vi "Behavior.vi"() -> ()   [LabVIEW 2014]
doc: "Use this template to measure or generate signals using the DAQ Assistant Express VI and NI-DAQmx. Double click the DAQ Assistant Express VI to launch a configuration wizard which steps you through configuring a measurement or generation.\n\nNote: You must have an NI-DAQmx compatible device installed to use this Express VI. Refer to the DAQ Quick Start Guide for NI-DAQ 7.0 for a list of compatible devices."
uses:
  <vilib>/userdefined/High Color/IMAQdx.ctl
  QuadraturePositionDecoder/QuadraturePositionDecoder.lvclass
  Imaging/Imaging.lvclass
  Photodiode/Photodiode.lvclass
panel:
  in  "Analog Signals":bool=TRUE
  in  "Ball Motion":bool=TRUE
  in  "Video":bool=TRUE
  in  "Base path":path
  out "Waveform Chart":dynamicdata(graph)
  in  "Remote":bool
  out "Scanning":bool
  out "Recording":bool
  out "File":path
  in  "Rec":bool
  out "File Path":path
  in  "Save Analog Signals":bool=TRUE
  out "Ball Position":u32
  in  "Compression":string(combo)="None"
  in  "Save Ball Motion":bool=TRUE
  in  "Save Video":bool=TRUE
  in  "Gain":dbl(slide)=2.6607250597988097 min=1.0 max=3.9810717055349722 scale=0.0..4.0
  in  "Exposure":dbl(slide)=16602.0 caption="Exposure Time" min=0.0 max=50000.0 scale=16.6..50000.0 scale format="%#_2p"
  out "FPS":dbl format="%#.0f"
  in  "Fps":i32=20
  out "Video Frames":T1(plugin-control)
  out "Ball Speed":dbl(graph)
  out "Stopped":bool
  in  "Stop":bool
  # "TODO:\n1. Make EyeParams me properly set\n2. Synchronization"
  # "Hardware Used For Quadrature Decoding"
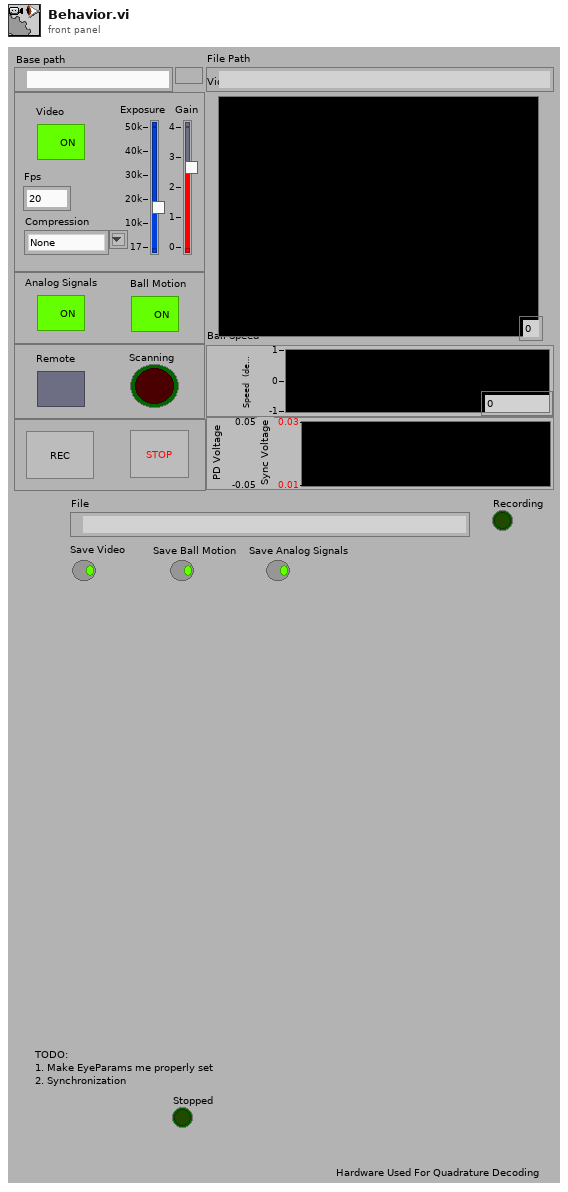
[diagram p1: front panel]
types:
  T1 = typedef "IMAQ Image.ctl" = refnum<image>
  T2 = typedef "IMAQdx.ctl" = refnum<k21>
  T3 = cluster{"VISA resource name":refnum<visa-resource-name>, "Counter":tag, "A Input Terminal":tag, "B Input Terminal":tag, "Z Index Terminal":tag, "Camera Name":T2, "Timestamp Counter":tag, "Timestamp Source":tag, "photodiode":tag, "scanimageframesync":tag, "Default Path":string}[]
  T4 = cluster{"VISA resource name":refnum<visa-resource-name>, "Counter":tag, "A Input Terminal":tag, "B Input Terminal":tag, "Z Index Terminal":tag, "Camera Name":T2, "Timestamp Counter":tag, "Timestamp Source":tag, "photodiode":tag, "scanimageframesync":tag, "Default Path":string}
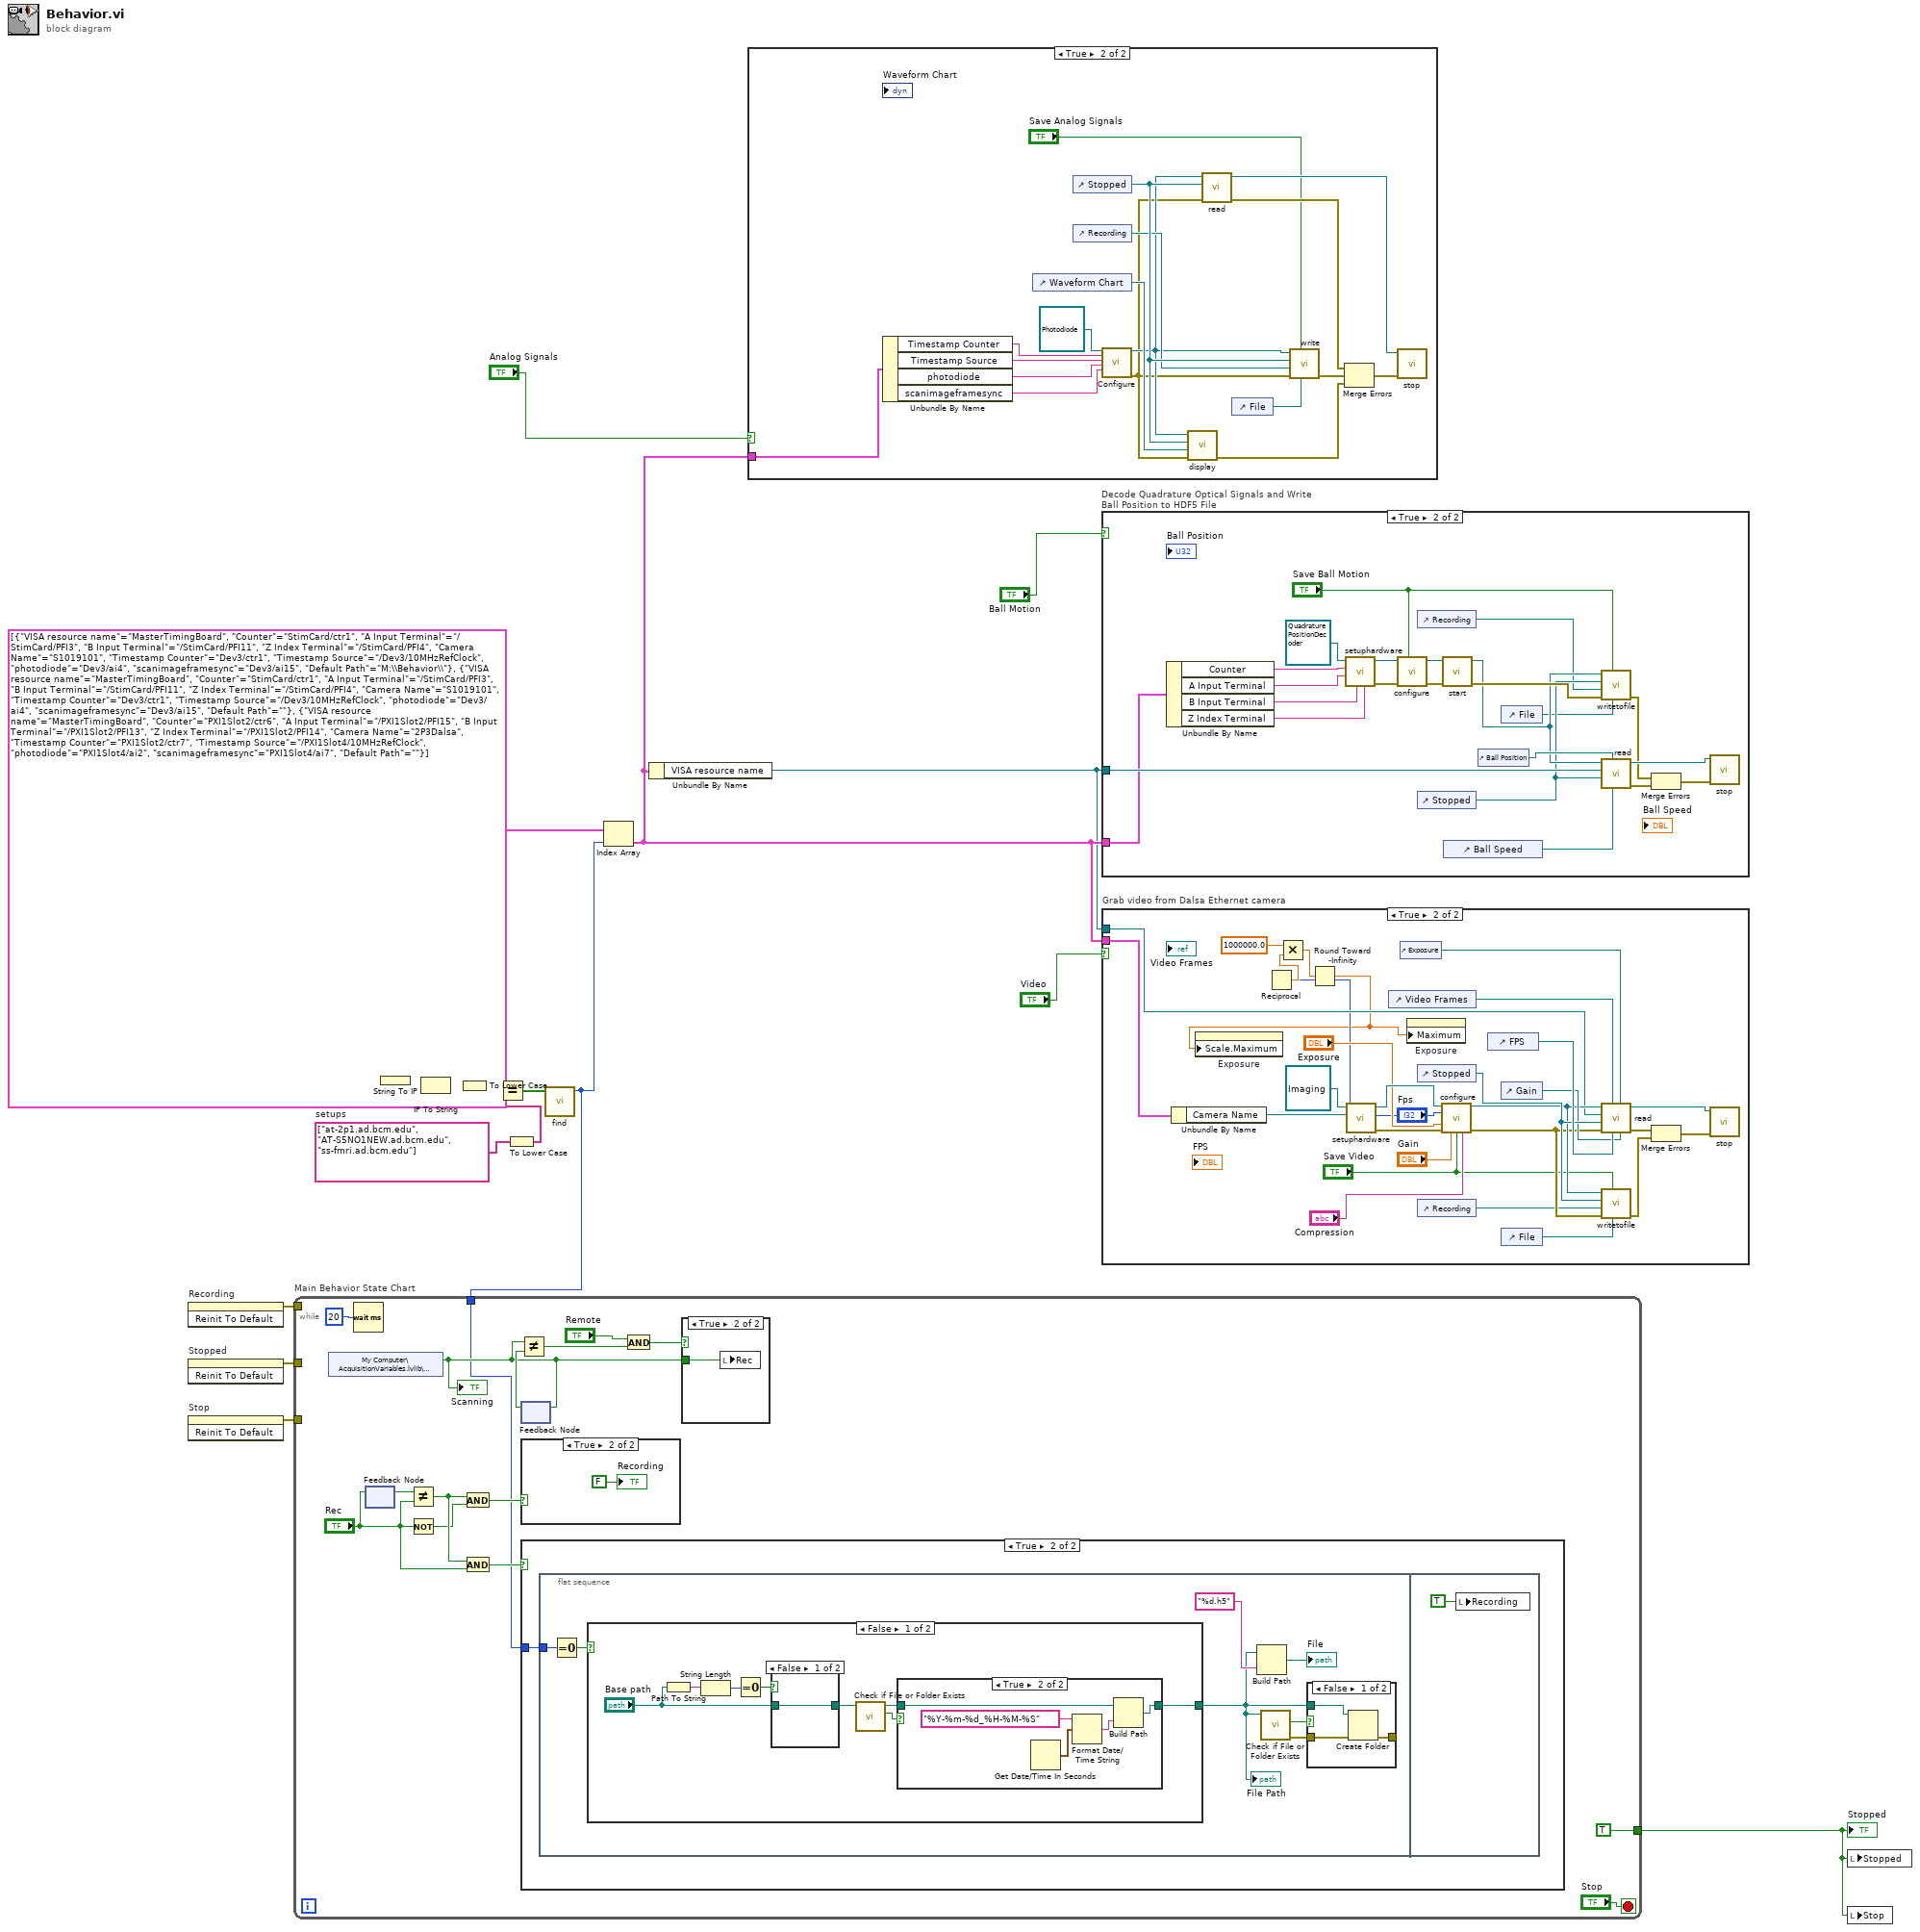
[diagram p0: block diagram]
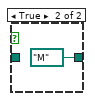
[diagram p8: hidden frame]
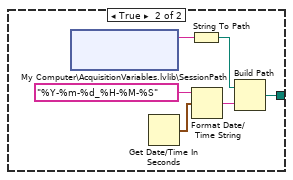
[diagram p10: hidden frame]
diagram:
  w3 = string[] ["at-2p1.ad.bcm.edu", "AT-S5NO1NEW.ad.bcm.edu", "ss-fmri.ad.bcm.edu"]  # setups
  n1 = invoke on="Recording" class="Bool (strict)" method="Reinit To Default"() -> (error out=w14:errorcluster)  [unwired: 3 in, 2 out]
  n2 = invoke on="Stopped" class="Bool (strict)" method="Reinit To Default"() -> (error out=w16:errorcluster)  [unwired: 3 in, 2 out]
  n3 = invoke on="Stop" class="Bool (strict)" method="Reinit To Default"() -> (error out=w17:errorcluster)  [unwired: 3 in, 2 out]
  n4 = String To IP() -> (0:w11:u32)  [unwired: 1 in]
  n5 = IP To String(2:w11) -> (0:w10:string)  [unwired: 1 in]
  n6 = To Lower Case(string=w10) -> (all lower case string=w9:string)
  n7 = To Lower Case(string=w3) -> (all lower case string=w2:string[])
  n8 = Equal?(x=w9, y=w2) -> (x = y?=w8:bool[])
  n9 = call "find.vi"("Array"=w8) -> ("Index"=w4:i32)  [unwired: 10 in]
  n10 = while "Main Behavior State Chart" {
    tunnel: [TRUE] -> w15
    tunnel: w17 -> [_]
    tunnel: w16 -> [_]
    tunnel: w14 -> [_]
    tunnel: w4 -> [w18]
    stop <- "Stop" stop-if-true
    n11 = shared-variable "My Computer\\AcquisitionVariables.lvlib\\AODScanning"() -> (w22:bool)  [unwired: 1 in, 1 out]
    "Scanning" <- w22
    n12 = Wait (ms)(milliseconds to wait=u32 20) -> ()  [unwired: 1 out]
    n13 = feedback-in #1("Rec") -> ()
    n14 = feedback #1() -> (w29:bool)  [unwired: 1 in]
    n15 = Not Equal?(x=w29, y="Rec") -> (x != y?=w27:bool)
    n16 = Not(x="Rec") -> (.not. x?=w26:bool)
    n17 = And(x=w27, y=w26) -> (x .and. y?=w24:bool)
    n18 = And(x=w27, y="Rec") -> (x .and. y?=w28:bool)
    n19 = feedback-in #2(w22) -> ()
    n20 = feedback #2() -> (w23:bool)  [unwired: 1 in]
    n21 = Not Equal?(x=w22, y=w23) -> (x != y?=w21:bool)
    n22 = case shown="True" w24 {
      frame False {
      }
      frame True {
        "Recording" <- FALSE
      }
    }
    n23 = case shown="True" w28 {
      tunnel: w18 -> [_ w35]
      frame False {
      }
      frame True {
        n24 = flat-sequence {
          tunnel: w35 -> [w38]
          frame #0 {
            n25 = Equal To 0?(x=w38) -> (x = 0?=w37:bool)
            n26 = case shown="False" w37 {
              tunnel: [w48 w60] -> w36
              frame False {
                n27 = Path To String(path="Base path") -> (string=w47:string)
                n28 = String Length(string=w47) -> (length=w46:i32)
                n29 = Equal To 0?(x=w46) -> (x = 0?=w45:bool)
                n30 = case shown="False" w45 {
                  tunnel: "Base path" -> [w51 _]
                  tunnel: [w51 path "M:/" ("Base path")] -> w43
                  frame False {
                  }
                  frame True {
                  }
                }
                n31 = call <vilib>:"Check if File or Folder Exists.vi"("path"=w43) -> ("file or folder exists?"=w49:bool, "dup path"=w50:path)  [unwired: 8 in, 1 out]
                n32 = case shown="True" w49 {
                  tunnel: w50 -> [w53 w56]
                  tunnel: [w53 w55] -> w48
                  frame False {
                  }
                  frame True {
                    n33 = Get Date/Time In Seconds() -> (seconds since 1Jan1904=w57:timestamp)
                    n34 = Format Date/Time String(time format string (%c)="%Y-%m-%d_%H-%M-%S", seconds (now)=w57) -> (date/time string=w58:string)  [unwired: 1 out]
                    n35 = Build Path(base path=w56, name or relative path=w58) -> (appended path=w55:path)
                  }
                }
              }
              frame True {
                n36 = shared-variable "My Computer\\AcquisitionVariables.lvlib\\SessionPath"() -> (w64:string)  [unwired: 2 in, 3 out]
                n37 = Get Date/Time In Seconds() -> (seconds since 1Jan1904=w63:timestamp)
                n38 = String To Path(string=w64) -> (path=w61:path)
                n39 = Format Date/Time String(time format string (%c)="%Y-%m-%d_%H-%M-%S", seconds (now)=w63) -> (date/time string=w62:string)  [unwired: 1 out]
                n40 = Build Path(base path=w61, name or relative path=w62) -> (appended path=w60:path)
              }
            }
            "File Path" <- w36
            n41 = Build Path(base path=w36, name or relative path="%d.h5" ("string")) -> (appended path=→"File":path)
            n42 = call <vilib>:"Check if File or Folder Exists.vi"("path"=w36) -> ("error out"=w40:errorcluster, "file or folder exists?"=w39:bool)  [unwired: 8 in, 1 out]
            n43 = case shown="False" w39 {
              tunnel: w36 -> [w67 _]
              tunnel: w40 -> [w66 w68]
              tunnel: [w65 w68] -> _
              frame False {
                n44 = Create Folder(path (use dialog)=w67, error in=w66) -> (error out=w65:errorcluster)  [unwired: 1 in, 2 out]
              }
              frame True {
              }
            }
          }
          frame #1 {
            n45 = local write "Recording"(TRUE) -> ()
          }
        }
      }
    }
    n46 = And(x="Remote", y=w21) -> (x .and. y?=w19:bool)
    n47 = case shown="True" w19 {
      tunnel: w22 -> [_ w33]
      frame False {
      }
      frame True {
        n48 = local write "Rec"(w33) -> ()
      }
    }
  }
  "Stopped" <- w15
  n49 = Index Array(array=T3 [{"VISA resource name"="MasterTimingBoard", "Counter"="StimCard/ctr1", "A Input Terminal"="/StimCard/PFI3", "B Input Terminal"="/StimCard/PFI11", "Z Index Terminal"="/StimCard/PFI4", "Camera Name"="S1019101", "Timestamp Counter"="Dev3/ctr1", "Timestamp Source"="/Dev3/10MHzRefClock", "photodiode"="Dev3/ai4", "scanimageframesync"="Dev3/ai15", "Default Path"="M:\\Behavior\\"}, {"VISA resource name"="MasterTimingBoard", "Counter"="StimCard/ctr1", "A Input Terminal"="/StimCard/PFI3", "B Input Terminal"="/StimCard/PFI11", "Z Index Terminal"="/StimCard/PFI4", "Camera Name"="S1019101", "Timestamp Counter"="Dev3/ctr1", "Timestamp Source"="/Dev3/10MHzRefClock", "photodiode"="Dev3/ai4", "scanimageframesync"="Dev3/ai15", "Default Path"=""}, {"VISA resource name"="MasterTimingBoard", "Counter"="PXI1Slot2/ctr6", "A Input Terminal"="/PXI1Slot2/PFI15", "B Input Terminal"="/PXI1Slot2/PFI13", "Z Index Terminal"="/PXI1Slot2/PFI14", "Camera Name"="2P3Dalsa", "Timestamp Counter"="PXI1Slot2/ctr7", "Timestamp Source"="/PXI1Slot4/10MHzRefClock", "photodiode"="PXI1Slot4/ai2", "scanimageframesync"="PXI1Slot4/ai7", "Default Path"=""}], index=w4) -> (element=w12:T4)
  n50 = Unbundle By Name(w12) -> ("VISA resource name"=w1:refnum<visa-resource-name>)
  n51 = case shown="True" "Analog Signals" {
    tunnel: w12 -> [_ w74]
    frame False {
    }
    frame True {
      n52 = Unbundle By Name(w74) -> ("Timestamp Counter"=w73:tag, "Timestamp Source"=w72:tag, "photodiode"=w71:tag, "scanimageframesync"=w70:tag)
      n53 = control-ref of="Waveform Chart"() -> (w78:refnum<vi>)
      n54 = control-ref of="Stopped"() -> (w86:refnum<vi>)
      n55 = control-ref of="Recording"() -> (w79:refnum<vi>)
      n56 = call-dynamic "Configure.vi"("Photodiode in"=refnum<class "Photodiode.lvclass"> refnum ("Photodiode.lvclass"), "Timestamp Counter"=w73, "Timestamp Source"=w72, "photodiode"=w71, "scanimageframesync"=w70) -> ("Photodiode out"=w76:refnum<class "Photodiode.lvclass">, "error out"=w75:errorcluster)  [unwired: 13 in]
      n57 = call-dynamic "display.vi"("error in (no error)"=w75, "PD  Display"=w78, "Stop Flag Reference"=w86, "Photodiode in"=w76) -> ("error out"=w83:errorcluster)  [unwired: 4 in, 3 out]
      n58 = call-dynamic "read.vi"("error in (no error)"=w75, "Stop Flag Reference"=w86, "Photodiode in"=w76) -> ("error out"=w84:errorcluster, "Photodiode out"=w87:refnum<class "Photodiode.lvclass">)  [unwired: 7 in]
      n59 = control-ref of="File"() -> (w80:refnum<vi>)
      n60 = call-dynamic "write.vi"("FilePath"=w80, "Save Analog Signals"="Save Analog Signals", "error in (no error)"=w75, "Rec Flag Reference"=w79, "Stop Flag Reference"=w86, "Photodiode in"=w76) -> ("error out"=w81:errorcluster)  [unwired: 4 in, 1 out]
      n61 = Merge Errors(w84, w81, w83) -> (w85:errorcluster)
      n62 = call-dynamic "stop.vi"("error in (no error)"=w85, "Photodiode in"=w87) -> ()  [unwired: 8 in, 2 out]
    }
  }
  n63 = case "Decode Quadrature Optical Signals and Write Ball Position to HDF5 File" shown="True" "Ball Motion" {
    tunnel: w1 -> [_ w97]
    tunnel: w12 -> [_ w92]
    frame False {
    }
    frame True {
      n64 = Unbundle By Name(w92) -> ("Counter"=w91:tag, "A Input Terminal"=w90:tag, "B Input Terminal"=w89:tag, "Z Index Terminal"=w88:tag)
      n65 = call-dynamic "setuphardware.vi"("Z Index Terminal"=w88, "B Input Terminal"=w89, "A Input Terminal"=w90, "Counter"=w91, "QuadraturePositionDecoder in"=refnum<class "QuadraturePositionDecoder.lvclass"> refnum ("QuadraturePositionDecoder.lvclass")) -> ("error out"=w108:errorcluster, "QuadraturePositionDecoder out"=w109:refnum<class "QuadraturePositionDecoder.lvclass">)  [unwired: 5 in]
      n66 = call-dynamic "configure.vi"("Save Data"="Save Ball Motion", "error in (no error)"=w108, "QuadraturePositionDecoder in"=w109) -> ("error out"=w106:errorcluster, "QuadraturePositionDecoder out"=w107:refnum<class "QuadraturePositionDecoder.lvclass">)  [unwired: 7 in]
      n67 = control-ref of="Recording"() -> (w93:refnum<vi>)
      n68 = control-ref of="Stopped"() -> (w96:refnum<vi>)
      n69 = call-dynamic "start.vi"("error in (no error)"=w106, "QuadraturePositionDecoder in"=w107) -> ("error out"=w102:errorcluster, "QuadraturePositionDecoder out"=w101:refnum<class "QuadraturePositionDecoder.lvclass">)  [unwired: 8 in]
      n70 = control-ref of="Ball Speed"() -> (w103:refnum<vi>)
      n71 = control-ref of="Ball Position"() -> (w105:refnum<vi>)
      n72 = control-ref of="File"() -> (w94:refnum<vi>)
      n73 = call-dynamic "writetofile.vi"("FilePath"=w94, "Save Ball Motion"="Save Ball Motion", "error in (no error)"=w102, "Rec Flag Reference"=w93, "Stop Flag Reference"=w96, "QuadraturePositionDecoder in"=w101) -> ("error out"=w100:errorcluster)  [unwired: 4 in, 1 out]
      n74 = call-dynamic "read.vi"("Current Speed"=w103, "Current Position"=w105, "Stop Flag Reference"=w96, "VISA resource name"=w97, "QuadraturePositionDecoder in"=w101) -> ("error out"=w99:errorcluster, "QuadraturePositionDecoder out"=w104:refnum<class "QuadraturePositionDecoder.lvclass">)  [unwired: 5 in]
      n75 = Merge Errors(w100, w99) -> (w98:errorcluster)
      n76 = call-dynamic "stop.vi"("error in (no error)"=w98, "QuadraturePositionDecoder in"=w104) -> ()  [unwired: 8 in, 2 out]
    }
  }
  n77 = case "Grab video from Dalsa Ethernet camera" shown="True" "Video" {
    tunnel: w1 -> [_ w122]
    tunnel: w12 -> [_ w118]
    frame False {
    }
    frame True {
      n78 = Unbundle By Name(w118) -> ("Camera Name"=w117:T2)
      n79 = Reciprocal(x="Fps") -> (1/x=w115:dbl)
      n80 = Multiply(x=1000000.0, y=w115) -> (x*y=w113:dbl)
      n81 = Round Toward -Infinity(1:w113) -> (0:w111:dbl)
      n82 = property on="Exposure" class="Slide (strict)"("Scale.Maximum"=w111) -> ()  [unwired: 2 in, 2 out]
      n83 = call-dynamic "setuphardware.vi"("Camera Name"=w117, "Imaging in"=refnum<class "Imaging.lvclass"> refnum ("Imaging.lvclass")) -> ("error out"=w124:errorcluster, "Imaging out"=w125:refnum<class "Imaging.lvclass">)  [unwired: 8 in]
      n84 = control-ref of="Video Frames"() -> (w136:refnum<vi>)
      n85 = control-ref of="Exposure"() -> (w130:refnum<vi>)
      n86 = property on="Exposure" class="Slide (strict)"("Maximum"=w111) -> ()  [unwired: 2 in, 2 out]
      n87 = control-ref of="Stopped"() -> (w132:refnum<vi>)
      n88 = control-ref of="Recording"() -> (w119:refnum<vi>)
      n89 = call-dynamic "configure.vi"("Imaging in"=w125, "Frame Rate"="Fps", "Exposure"="Exposure", "error in (no error)"=w124, "Gain"="Gain", "Save Data"="Save Video", "Codec"="Compression") -> ("Imaging out"=w128:refnum<class "Imaging.lvclass">, "error out"=w127:errorcluster)  [unwired: 7 in]
      n90 = control-ref of="FPS"() -> (w135:refnum<vi>)
      n91 = control-ref of="Gain"() -> (w129:refnum<vi>)
      n92 = control-ref of="File"() -> (w121:refnum<vi>)
      n93 = call-dynamic "read.vi"("Gain"=w129, "Exposure"=w130, "Actual Rate"=w135, "Video Display"=w136, "error in"=w127, "Stop Flag Reference"=w132, "VISA resource name"=w122, "Imaging in"=w128) -> ("error out"=w134:errorcluster, "Imaging out"=w137:refnum<class "Imaging.lvclass">)  [unwired: 2 in]
      n94 = call-dynamic "writetofile.vi"("FilePath"=w121, "Save Video"="Save Video", "error in (no error)"=w127, "Rec Flag Reference"=w119, "Stop Flag Reference"=w132, "Imaging in"=w128) -> ("error out"=w133:errorcluster)  [unwired: 4 in, 1 out]
      n95 = Merge Errors(w134, w133) -> (w131:errorcluster)
      n96 = call-dynamic "stop.vi"("error in (no error)"=w131, "Imaging in"=w137) -> ()  [unwired: 8 in, 2 out]
    }
  }
  n97 = local write "Stopped"(w15) -> ()
  n98 = local write "Stop"(w15) -> ()
